vi "max_min.vi"(2 "B":dbl, 3 "A":dbl) -> (0 "MIN":dbl, 1 "MAX":dbl)   [LabVIEW 2009]
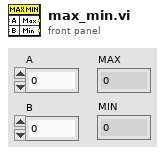
[diagram p1: front panel]
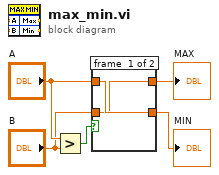
[diagram p0: block diagram]
diagram:
  n1 = Greater?(x="A", y="B") -> (0:w5:bool)
  n2 = case shown="True" w5 {
    tunnel: "A" -> [w7 w9]
    tunnel: "B" -> [w6 w8]
    tunnel: [w6 w9] -> w2
    tunnel: [w7 w8] -> w1
    frame #0 {
    }
    frame #1 {
    }
  }
  "MAX" <- w2
  "MIN" <- w1
